vi "setRange.vi"(8 "error in (no error)":errorcluster, 10 "Range":dbl format="%#_10g", 11 "Electrometer in":refnum<class "Electrometer.lvclass">) -> (0 "error out":errorcluster, 3 "Electrometer out":refnum<class "Electrometer.lvclass">)   [LabVIEW 2016, in "Electrometer.lvclass"]
uses:
  Electrometer.lvclass
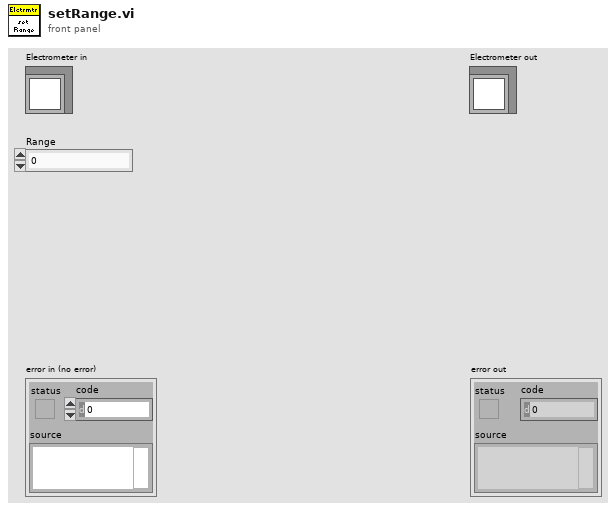
[diagram p1: front panel]
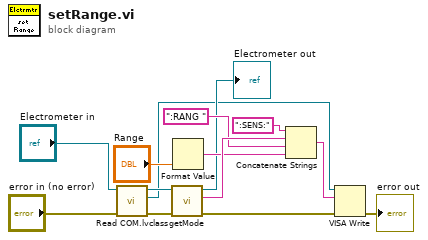
[diagram p0: block diagram]
diagram:
  n1 = call "Read COM.lvclass.vi"("error in (no error)"="error in (no error)", "Electrometer in"="Electrometer in") -> ("error out"=w11:errorcluster, "VISA"=w4:refnum<visa-resource-name>, "Electrometer out"=w12:refnum<class "Electrometer.lvclass">)  [unwired: 7 in]
  n2 = call "getMode.vi"("error in (no error)"=w11, "Electrometer in"=w12) -> ("error out"=w2:errorcluster, "Mode"=w9:string, "Electrometer out"=→"Electrometer out":refnum<class "Electrometer.lvclass">)  [unwired: 7 in]
  n3 = Format Value(value (0)="Range") -> (output string=w6:string)  [unwired: 2 in]
  n4 = Concatenate Strings(":SENS:", w9, ":RANG " ("string"), w6) -> (w3:string)
  n5 = VISA Write(VISA resource name=w4, write buffer=w3, error in (no error)=w2) -> (error out=→"error out":errorcluster)  [unwired: 2 out]
